vi "AlternatingLEDs.vi"() -> ()   [LabVIEW 2015]
doc: "Tab selector allows user to utilize two modes:\n\n\"Alternating\" continuously alternately lights hardware LEDs until the front-panel Stop Button is clicked.\n\"Toggled\" alternately lights the front-panel LED indicators until Stop Button is clicked."
panel:
  in  "Tab Control":enum32{"Alternating", "Toggled"}(tab)
  in  "stop":bool
  out "LED 2":bool
  out "LED 1":bool
  in  "stop 2":bool
  in  "Boolean":bool
  out "LED 3":bool
  out "LED 4":bool
  # "Alternates hardware LED until stopped"
  # "Toggles LEDs using switch"
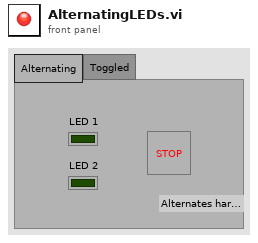
[diagram p1: front panel]
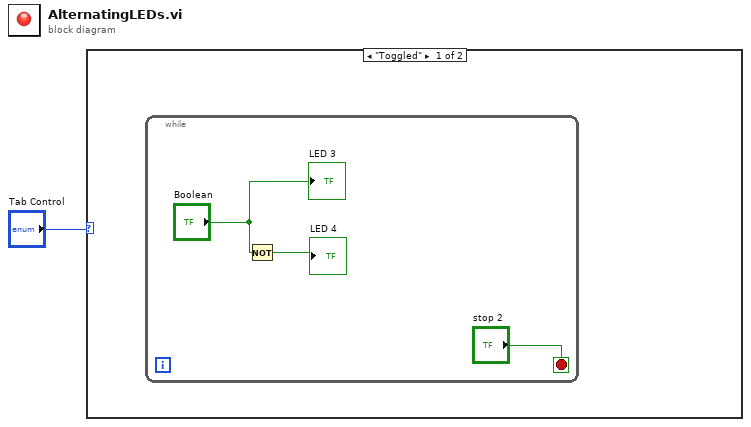
[diagram p0: block diagram]
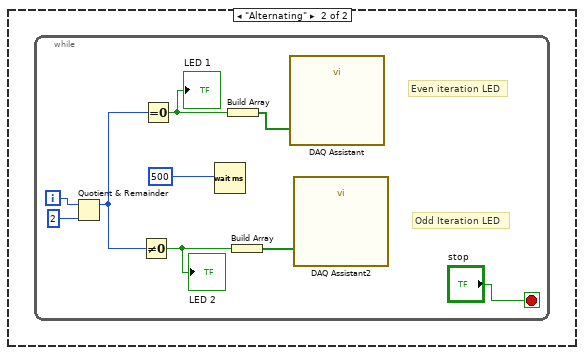
[diagram p2: hidden frame]
diagram:
  n1 = case shown="\"Toggled\"" "Tab Control" {
    frame "Toggled" {
      n2 = while {
        stop <- "stop 2" stop-if-true
        n3 = Not(x="Boolean") -> (.not. x?=→"LED 4":bool)
        "LED 3" <- "Boolean"
      }
    }
    frame "Alternating" {
      n4 = while {
        i -> [w13]
        stop <- "stop" stop-if-true
        # "Odd Iteration LED"
        # "Even iteration LED"
        n5 = Quotient & Remainder(x=w13, y=2) -> (x-y*floor(x/y)=w9:i32)  [unwired: 1 out]
        n6 = Not Equal To 0?(x=w9) -> (x != 0?=w7:bool)
        "LED 2" <- w7
        n7 = Equal To 0?(x=w9) -> (x = 0?=w8:bool)
        "LED 1" <- w8
        n8 = Wait (ms)(milliseconds to wait=u32 500) -> ()  [unwired: 1 out]
        n9 = Build Array(w8) -> (w6:bool[])
        n10 = Build Array(w7) -> (w5:bool[])
        n11 = call "DAQ Assistant"("data"=w6) -> ()  [unwired: 17 in, 2 out]
        n12 = call "DAQ Assistant2"("data"=w5) -> ()  [unwired: 17 in, 2 out]
      }
    }
  }
